vi "Footer.vi"() -> ()   [LabVIEW 2011]
uses:
  <vilib>/Utility/miscctls.llb/LVPointTypeDef.ctl
  Globals/Global VI.vi
panel:
  in  "Last Button":bool
  in  "Next Button":bool
  in  "First Button":bool
  in  "Previous Button":bool
  in  "Cluster":T1
  out "array":bool[](array[boolean])
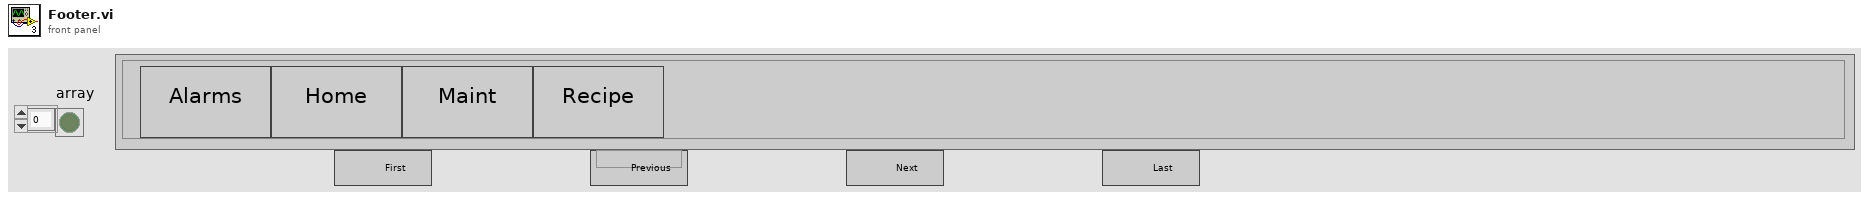
[diagram p1: front panel]
types:
  T1 = cluster{"OK Button":bool, "OK Button 2":bool, "OK Button 3":bool, "OK Button 4":bool, "OK Button 5":bool, "OK Button 6":bool, "OK Button 7":bool, "OK Button 8":bool, "OK Button 9":bool, "OK Button 10":bool, "OK Button 11":bool, "OK Button 12":bool, "OK Button 13":bool}
  T2 = typedef "LVPointTypeDef.ctl" = cluster{"Horizontal":i16, "Vertical":i16}
  T3 = enum16{"Always On", "Always Off", "Off While Running"}
  T4 = typedef "LVRectTypeDef.ctl" = cluster{"left":i16, "top":i16, "right":i16, "bottom":i16}
  T5 = typedef "LVAllMonitorsDisplayTypeDef.ctl" = cluster{"Bounds":cluster{"Left":i16, "Top":i16, "Right":i16, "Bottom":i16}, "Depth":i16}[]
  T6 = cluster{"Bounds":cluster{"Left":i16, "Top":i16, "Right":i16, "Bottom":i16}, "Depth":i16}
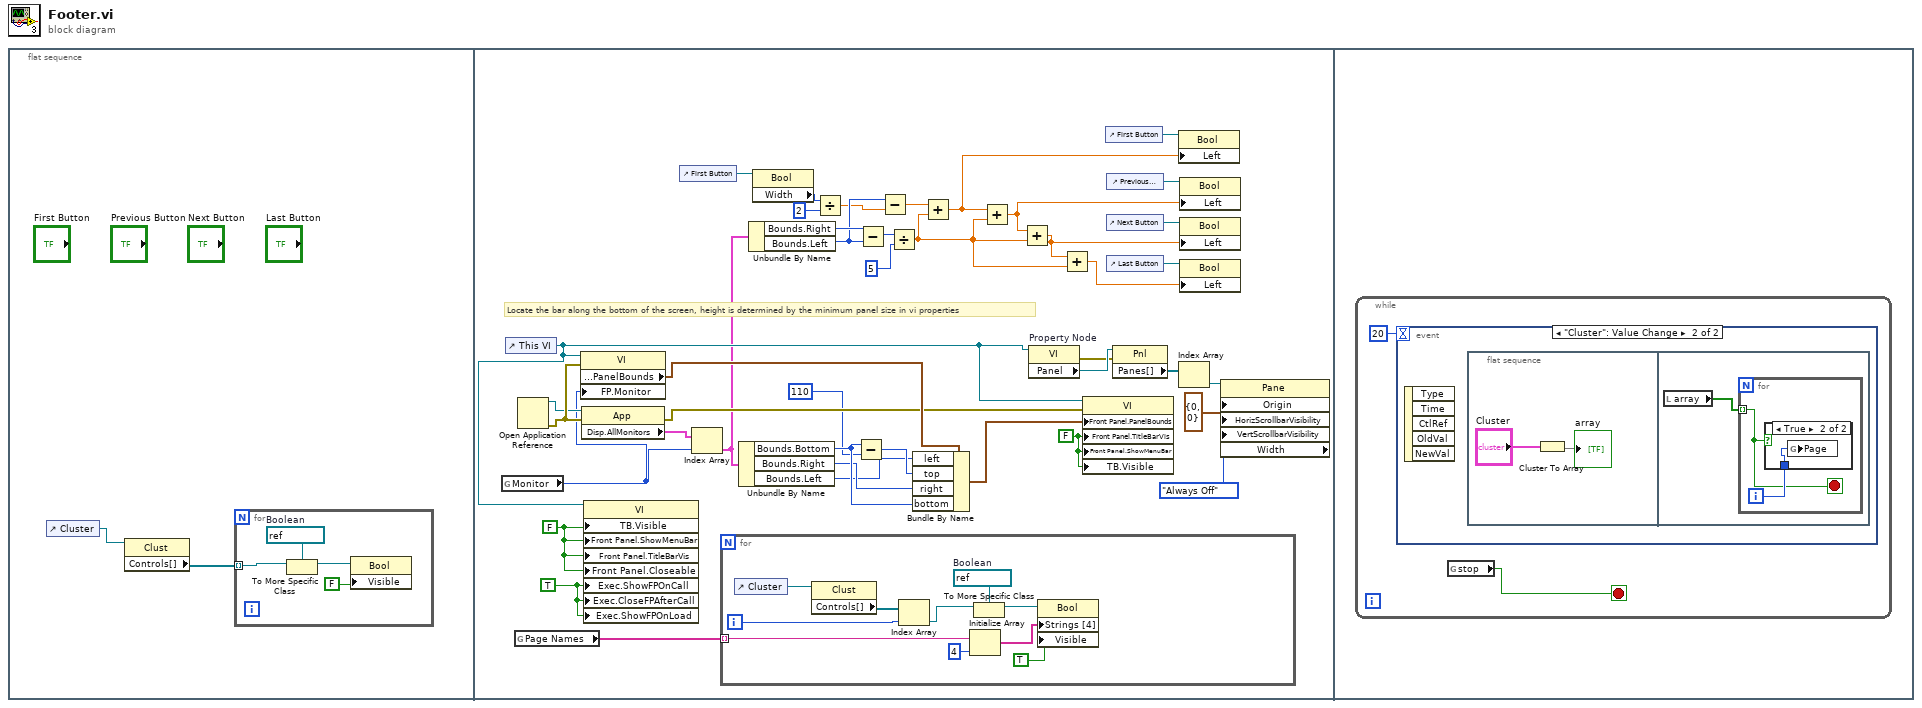
[diagram p0: block diagram]
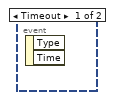
[diagram p2: hidden frame]
diagram:
  n1 = flat-sequence {
    frame #0 {
      n2 = control-ref of="Cluster"() -> (w1:refnum<vi>)
      n3 = property class="Clust"(reference=w1) -> ("Controls[]"=w2:refnum<vi>[])  [unwired: 1 in, 2 out]
      n4 = for {
        tunnel: w2 -> [w3] mode=indexing
        w4 = refnum<vi> refnum  # Boolean
        n5 = To More Specific Class(target class=w4, reference=w3) -> (specific class reference=w5:refnum<vi>)  [unwired: 1 in, 1 out]
        n6 = property class="Bool"(reference=w5, "Visible"=FALSE) -> ()  [unwired: 1 in, 2 out]
      }
    }
    frame #1 {
      w30 = TRUE ("Execution:Show Front Panel On Call")
      w29 = FALSE ("Tool Bar:Visible")
      w31 = T3."Always Off" ("Horizontal Scrollbar Visibility")
      w34 = FALSE ("Front Panel Window:Title Bar Visible")
      # "Locate the bar along the bottom of the screen, height is determined by the minimum panel size in vi properties"
      n7 = global read "Global VI.vi" "Monitor"() -> (w32:u16)
      n8 = control-ref of="This VI"() -> (w28:refnum<vi>)
      n9 = global read "Global VI.vi" "Page Names"() -> (w33:string[])
      n10 = Open Application Reference() -> (0:w48:errorcluster, 3:w47:refnum<vi>)  [unwired: 4 in]
      n11 = property class="VI"(reference=w28, error in=w48, "FP.Monitor"=w32) -> ("Front Panel.PanelBounds"=w44:T4)  [unwired: 2 out]
      n12 = property class="App"(reference=w47, error in=w48) -> (error out=w42:errorcluster, "Disp.AllMonitors"=w41:T5)  [unwired: 1 out]
      n13 = property class="VI"(reference=w28, "TB.Visible"=w29, "Front Panel.ShowMenuBar"=w29, "Front Panel.TitleBarVis"=w29, "Front Panel.Closeable"=w29, "Exec.ShowFPOnCall"=w30, "Exec.CloseFPAfterCall"=w30, "Exec.ShowFPOnLoad"=w30) -> ()  [unwired: 1 in, 2 out]
      n14 = control-ref of="First Button"() -> (w12:refnum<vi>)
      n15 = Index Array(array=w41, index=w32) -> (element=w21:T6)
      n16 = for {
        tunnel: w33 -> [w58] mode=indexing
        i -> [w51]
        w57 = refnum<vi> refnum  # Boolean
        n17 = control-ref of="Cluster"() -> (w49:refnum<vi>)
        n18 = property class="Clust"(reference=w49) -> ("Controls[]"=w53:refnum<vi>[])  [unwired: 1 in, 2 out]
        n19 = Index Array(array=w53, index=w51) -> (element=w52:refnum<vi>)
        n20 = Initialize Array(w58, 4 ("dimension size")) -> (w54:string[])
        n21 = To More Specific Class(target class=w57, reference=w52) -> (specific class reference=w56:refnum<vi>)  [unwired: 1 in, 1 out]
        n22 = property class="Bool"(reference=w56, "Strings [4]"=w54, "Visible"=TRUE) -> ()  [unwired: 1 in, 2 out]
      }
      n23 = Unbundle By Name(w21) -> ("Bounds.Bottom"=w46:i16, "Bounds.Right"=w27:i16, "Bounds.Left"=w26:i16)
      n24 = Unbundle By Name(w21) -> ("Bounds.Right"=w20:i16, "Bounds.Left"=w9:i16)
      n25 = property class="Bool"(reference=w12) -> ("Width"=w11:u32)  [unwired: 1 in, 2 out]
      n26 = Divide(x=w11, y=u32 2) -> (x/y=w8:dbl)
      n27 = Subtract(x=w46, y=i16 110) -> (x-y=w45:i16)
      n28 = Subtract(x=w20, y=w9) -> (x-y=w19:i16)
      n29 = Subtract(x=w9, y=w8) -> (x-y=w7:dbl)
      n30 = Divide(x=w19, y=i16 5) -> (x/y=w14:dbl)
      n31 = Bundle By Name(cluster=w44, "left"=w26, "top"=w45, "right"=w27, "bottom"=w46) -> (w43:T4)
      n32 = Add(x=w7, y=w14) -> (x+y=w17:dbl)
      n33 = Add(x=w17, y=w14) -> (x+y=w16:dbl)
      n34 = Add(x=w16, y=w14) -> (x+y=w15:dbl)
      n35 = property on="Property Node" class="VI"(reference=w28) -> (error out=w39:errorcluster, "Panel"=w40:refnum<vi>)  [unwired: 1 in, 1 out]
      n36 = Add(x=w15, y=w14) -> (x+y=w13:dbl)
      n37 = property class="VI"(reference=w28, error in=w42, "Front Panel.PanelBounds"=w43, "Front Panel.TitleBarVis"=w34, "Front Panel.ShowMenuBar"=w34, "TB.Visible"=w34) -> ()  [unwired: 2 out]
      n38 = control-ref of="First Button"() -> (w22:refnum<vi>)
      n39 = control-ref of="Previous Button"() -> (w23:refnum<vi>)
      n40 = control-ref of="Next Button"() -> (w24:refnum<vi>)
      n41 = control-ref of="Last Button"() -> (w25:refnum<vi>)
      n42 = property class="Pnl"(reference=w40, error in=w39) -> ("Panes[]"=w38:refnum<vi>[])  [unwired: 2 out]
      n43 = property class="Bool"(reference=w22, "Left"=w17) -> ()  [unwired: 1 in, 2 out]
      n44 = Index Array "Index Array"(array=w38) -> (element=w37:refnum<vi>)  [unwired: 1 in]
      n45 = property class="Bool"(reference=w23, "Left"=w16) -> ()  [unwired: 1 in, 2 out]
      n46 = property class="Bool"(reference=w24, "Left"=w15) -> ()  [unwired: 1 in, 2 out]
      n47 = property class="Bool"(reference=w25, "Left"=w13) -> ()  [unwired: 1 in, 2 out]
      n48 = property class="Pane" props=["Origin", "HorizScrollbarVisibility", "VertScrollbarVisibility", "Width"](reference=w37, "Origin"=T2 {"Horizontal"=0, "Vertical"=0}, "HorizScrollbarVisibility"=w31, "VertScrollbarVisibility"=w31) -> ()  [unwired: 1 in, 3 out]
    }
    frame #2 {
      n49 = while {
        stop <- w59 stop-if-true
        n50 = event shown="[1] \"Cluster\": Value Change" {
          selector: _ -> [_ _]
          dyn-events: _ -> [_ _]
          timeout: 20 -> [_ _]
          event Timeout {
            n51 = event-data() -> ()  [unwired: 1 in, 2 out]
          }
          event "Cluster": Value Change {
            n52 = event-data() -> ()  [unwired: 1 in, 5 out]
            n53 = flat-sequence {
              frame #0 {
                n54 = Cluster To Array(cluster="Cluster") -> (array=→"array":bool[])
              }
              frame #1 {
                n55 = local read "array"() -> (w63:bool[])
                n56 = for {
                  tunnel: w63 -> [w64] mode=indexing
                  i -> [w65]
                  stop <- w64 stop-if-true
                  n57 = case shown="True" w64 {
                    tunnel: w65 -> [_ w66]
                    frame False {
                    }
                    frame True {
                      n58 = global write "Global VI.vi" "Page"(w66) -> ()
                    }
                  }
                }
              }
            }
          }
        }
        n59 = global read "Global VI.vi" "stop"() -> (w59:bool)
      }
    }
  }
